vi "VISA shutter.vi"(8 "error in (no error)":errorcluster, 10 "button::shutter":bool, 11 "Cobolt in":refnum<class "Cobolt.lvclass">) -> (0 "error out":errorcluster, 3 "Cobolt out":refnum<class "Cobolt.lvclass">)   [LabVIEW 2012, in "Cobolt.lvclass"]
uses:
  Cobolt.lvclass
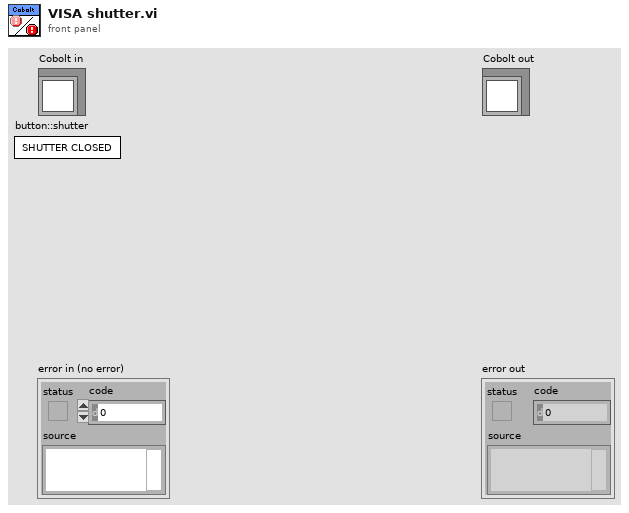
[diagram p1: front panel]
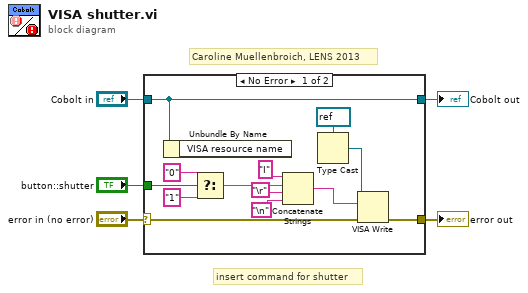
[diagram p0: block diagram]
diagram:
  # "insert command for shutter"
  # "Caroline Muellenbroich, LENS 2013"
  n1 = case shown="No Error" "error in (no error)" {
    selector: "error in (no error)" -> [w7 w20]
    tunnel: [w6 w20] -> w4
    tunnel: [w9 w19] -> w2
    tunnel: "Cobolt in" -> [w9 w19]
    tunnel: "button::shutter" -> [w8 _]
    frame No Error {
      n2 = Unbundle By Name(w9) -> ()  [unwired: 1 out]
      n3 = Select(t="0" ("string"), s=w8, f="1" ("string")) -> (s? t:f=w16:string)
      n4 = Concatenate Strings("I" ("string"), w16, "\r", "\n") -> (w17:string)
      n5 = Type Cast(type=refnum<visa-resource-name> refnum ("VISA resource name")) -> (*(type *) &x=w13:refnum<visa-resource-name>)  [unwired: 1 in]
      n6 = VISA Write(VISA resource name=w13, write buffer=w17, error in (no error)=w7) -> (error out=w6:errorcluster)  [unwired: 2 out]
    }
    frame Error {
    }
  }
  "error out" <- w4
  "Cobolt out" <- w2
